vi "sub_SDR_demod_QAM16.vi"(11 "Input Symbols":cdb[](array[numeric])) -> (3 "Array":bool[](array[boolean]))   [LabVIEW 2012]
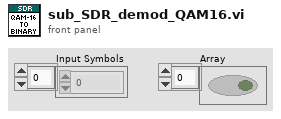
[diagram p1: front panel]
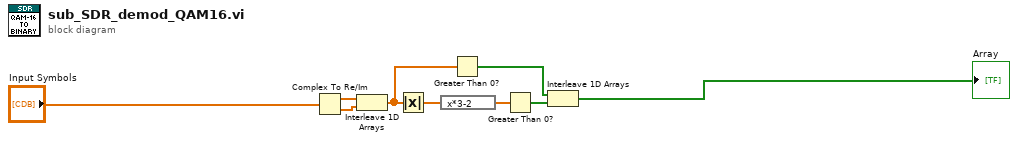
[diagram p0: block diagram]
diagram:
  n1 = Complex To Re/Im(x + iy="Input Symbols") -> (x=w1:dbl[], y=w2:dbl[])
  n2 = Interleave 1D Arrays(w1, w2) -> (w7:dbl[])
  n3 = Absolute Value(x=w7) -> (abs(x)=w4:dbl[])
  n4 = expression code="x*3-2"(w4) -> (w3:dbl[])
  n5 = Greater Than 0?(x=w7) -> (x > 0?=w5:bool[])
  n6 = Greater Than 0?(x=w3) -> (x > 0?=w6:bool[])
  n7 = Interleave 1D Arrays "Interleave 1D Arrays"(w5, w6) -> (→"Array":bool[])
